vi "Material-LoadSheet-Dialog.vi"(8 "error in":errorcluster, 11 "Material-RunTest.lvclass in":refnum<class "Material-RunTest.lvclass">) -> (0 "error out":errorcluster, 3 "Material-RunTest.lvclass out":refnum<class "Material-RunTest.lvclass">)   [LabVIEW 2013, in "Material-RunTest.lvclass"]
uses:
  Material-RunTest.lvclass
  Material-RunTest.lvclass/Material-RunTest.ctl
panel:
  in  "Help Button":bool
  in  "Last Sheet in lot":bool
  in  "Finished":bool
  out "String":string="Place the sheet of Material on the chuck now."
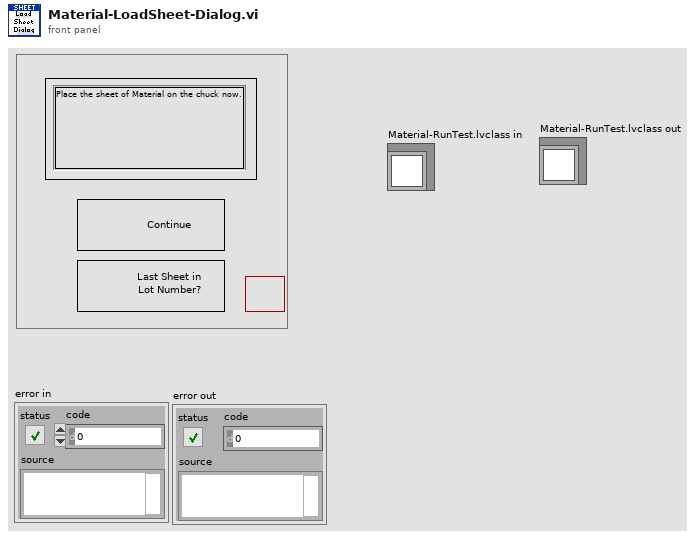
[diagram p1: front panel]
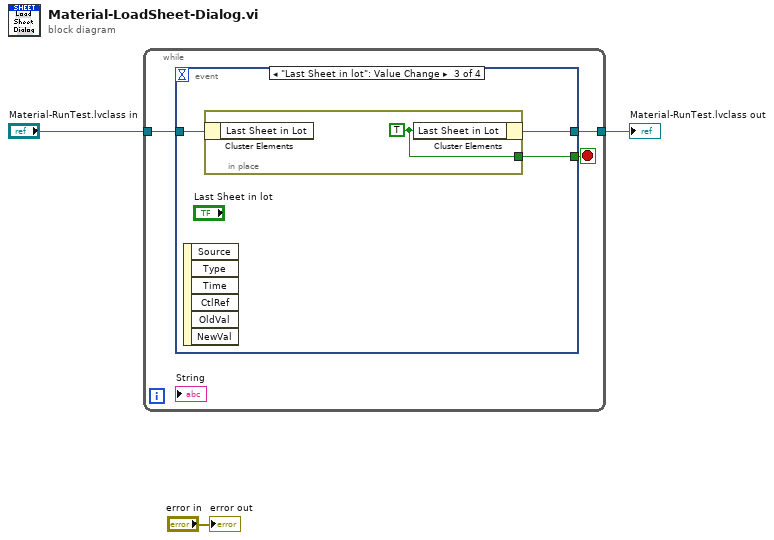
[diagram p0: block diagram]
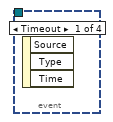
[diagram p2: hidden frame]
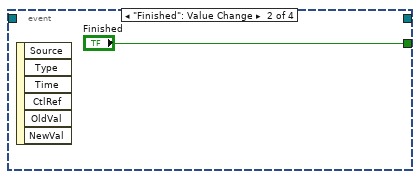
[diagram p3: hidden frame]
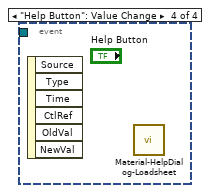
[diagram p4: hidden frame]
diagram:
  n1 = while {
    tunnel: "Material-RunTest.lvclass in" -> [w5]
    tunnel: [w4] -> w1
    stop <- w6 stop-if-true
    n2 = event shown="[2] \"Last Sheet in lot\": Value Change" {
      selector: _ -> [_ _ _ _]
      dyn-events: _ -> [_ _ _ _]
      timeout: _ -> [_ _ _ _]
      tunnel: [_ "Finished" w8 _] -> w6
      tunnel: w5 -> [_ _ w10 _]
      tunnel: [_ _ w9 _] -> w4
      event Timeout {
        n3 = event-data() -> ()  [unwired: 1 in, 3 out]
      }
      event "Finished": Value Change {
        n4 = event-data() -> ()  [unwired: 1 in, 6 out]
      }
      event "Last Sheet in lot": Value Change {
        n5 = event-data() -> ()  [unwired: 1 in, 6 out]
        n6 = in-place {
          in-place-border: [w11] -> w8
          w11 = TRUE ("Last Sheet in Lot")
          n7 = in-place-cluster #1(w10) -> ()  [unwired: 1 out]
          n8 = in-place-cluster #1("Last Sheet in Lot"=w11) -> (w9:refnum<class "Material-RunTest.lvclass">)
        }
      }
      event "Help Button": Value Change {
        n9 = event-data() -> ()  [unwired: 1 in, 6 out]
        n10 = call "Material-HelpDialog-Loadsheet.vi"() -> ()  [unwired: 12 in]
      }
    }
  }
  "Material-RunTest.lvclass out" <- w1
  "error out" <- "error in"
